vi "Write Communication.vi"(8 "error in (no error)":errorcluster, 10 "Communication":T1, 11 "SiemensDigitalEnergyMeter in":refnum<class "SiemensDigitalEnergyMeter.lvclass">) -> (0 "error out":errorcluster, 3 "SiemensDigitalEnergyMeter out":refnum<class "SiemensDigitalEnergyMeter.lvclass">)   [LabVIEW 2018, in "SensorPlugins.lvlib" / "SiemensDigitalEnergyMeter.lvclass"]
uses:
  SiemensDigitalEnergyMeter.lvclass
  TypeDefinitions/CommunicationControls.ctl
  <vilib>/Modbus/master/Modbus Master.lvclass
  <vilib>/Modbus/subvis/Transmission Data Unit (ADU)/IP Data Unit/IP Data Unit.lvclass
  <vilib>/Modbus/subvis/Protocol/TCP/TCP Master/TCP Master.lvclass
  SiemensDigitalEnergyMeter.lvclass/SiemensDigitalEnergyMeter.ctl
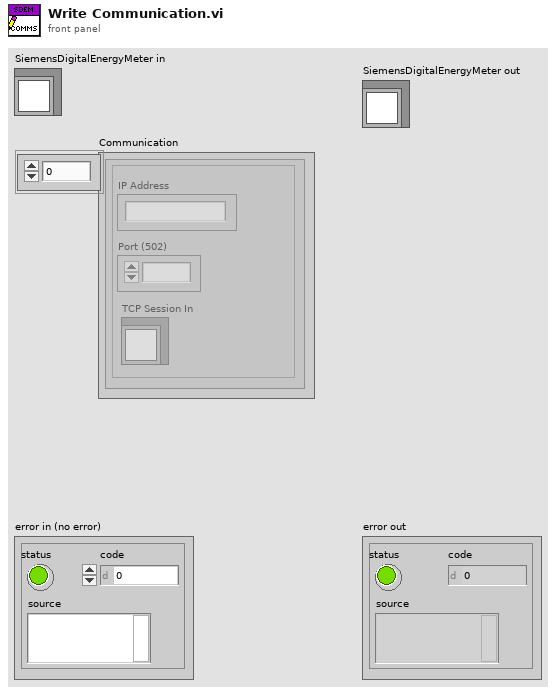
[diagram p1: front panel]
types:
  T1 = typedef "SensorPlugins.lvlib/SiemensDigitalEnergyMeter.lvclass/CommunicationControls.ctl" = cluster{"IP Address":string, "Port (502)":u16, "TCP Session In":refnum<class "Modbus Master.lvclass">}[]
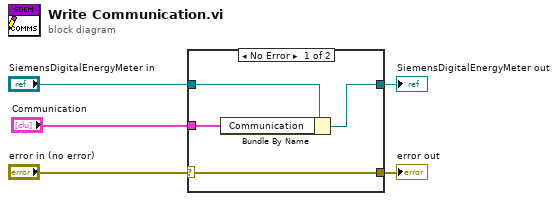
[diagram p0: block diagram]
diagram:
  n1 = case shown="No Error" "error in (no error)" {
    selector: "error in (no error)" -> [w9 w10]
    tunnel: [w9 w10] -> w4
    tunnel: [w7 w11] -> w2
    tunnel: "SiemensDigitalEnergyMeter in" -> [w8 w11]
    tunnel: "Communication" -> [w6 _]
    frame No Error {
      n2 = Bundle By Name(cluster=w8, "Communication"=w6) -> (w7:refnum<class "SiemensDigitalEnergyMeter.lvclass">)
    }
    frame Error {
    }
  }
  "error out" <- w4
  "SiemensDigitalEnergyMeter out" <- w2
